vi "Create Channel Buffer.vi"(8 "error in":errorcluster, 10 "Channel":string, 11 "BufferLossless in":refnum<class "BufferLossless.lvclass">) -> (0 "error out":errorcluster, 3 "BufferLossless out":refnum<class "BufferLossless.lvclass">)   [LabVIEW 2024, in "BufferLossless.lvclass"]
uses:
  BufferLossless.lvclass
  BufferLossless.lvclass/BufferLossless.ctl
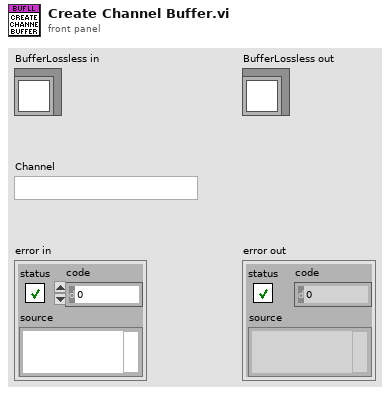
[diagram p1: front panel]
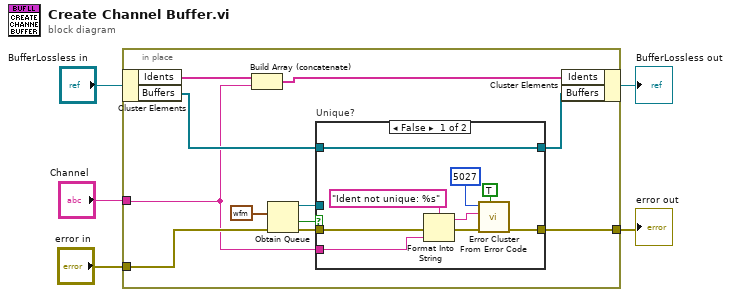
[diagram p0: block diagram]
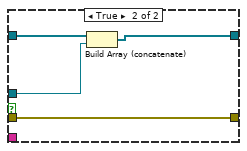
[diagram p2: hidden frame]
diagram:
  n1 = in-place {
    in-place-border: [w13] -> w1
    in-place-border: "Channel" -> [w9]
    in-place-border: "error in" -> [w16]
    n2 = in-place-cluster #1("BufferLossless in") -> ("Idents"=w10:string[], "Buffers"=w11:refnum<queue>[])
    n3 = Build Array (concatenate)(w10, w9) -> (w8:string[])
    n4 = Obtain Queue(element data type=waveform(dbl) {"t0"=timestamp(0 s since 1904-01-01), "dt"=1.0, "Y"=[]} ("Waveform"), error in (no error)=w16) -> (queue out=w6:refnum<queue>, created new?=w15:bool, error out=w14:errorcluster)  [unwired: 3 in]
    n5 = case "Unique?" shown="False" w15 {
      tunnel: w14 -> [w19 w29]
      tunnel: [w20 w29] -> w13
      tunnel: w9 -> [w18 _]
      tunnel: w11 -> [w17 w28]
      tunnel: w6 -> [_ w27]
      tunnel: [w17 w26] -> w7
      frame False {
        n6 = Format Into String(format string="Ident not unique: %s", error in=w19, w18) -> (resulting string=w21:string, error out=w23:errorcluster)  [unwired: 1 in]
        n7 = call <vilib>:"Error Cluster From Error Code.vi"("show call chain? (False)"=TRUE, "error in (no error)"=w23, "error message (\"\")"=w21, "error code (0)"=5027) -> ("error out"=w20:errorcluster)  [unwired: 5 in]
      }
      frame True {
        n8 = Build Array (concatenate)(w28, w27) -> (w26:refnum<queue>[])
      }
    }
    n9 = in-place-cluster #1("Idents"=w8, "Buffers"=w7) -> (→"BufferLossless out":refnum<class "BufferLossless.lvclass">)
  }
  "error out" <- w1
